vi "AddUser.vi"() -> ()   [LabVIEW 2020]
uses:
  <vilib>/Utility/error.llb/DialogType.ctl
  Global1.vi
  <vilib>/addons/database/Connection.llb/DB Tools Open Connec (String).vi
  <vilib>/addons/database/Connection.llb/Conn Execute.vi
  <vilib>/addons/database/Recordset.llb/Rec Destroy - Connection.vi
  <vilib>/addons/database/NI_Database_API.lvlib
panel:
  in  "员工编号":string
  in  "显示密码":bool
  in  "重复密码":string
  in  "权      限":enum16{"操作员", "管理员"}(ring)
  in  "取消":bool
  in  "确定":bool
  in  "密      码":string
  in  "用 户 名":string
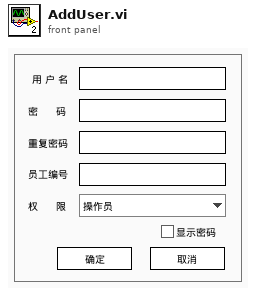
[diagram p1: front panel]
types:
  T1 = typedef "DialogType.ctl" = u16
  T2 = typedef "NI_Database_API.lvlib/Conn ObjectReference.ctl" = refnum<k1>
  T3 = typedef "NI_Database_API.lvlib/Rec ObjectReference.ctl" = refnum<k1>
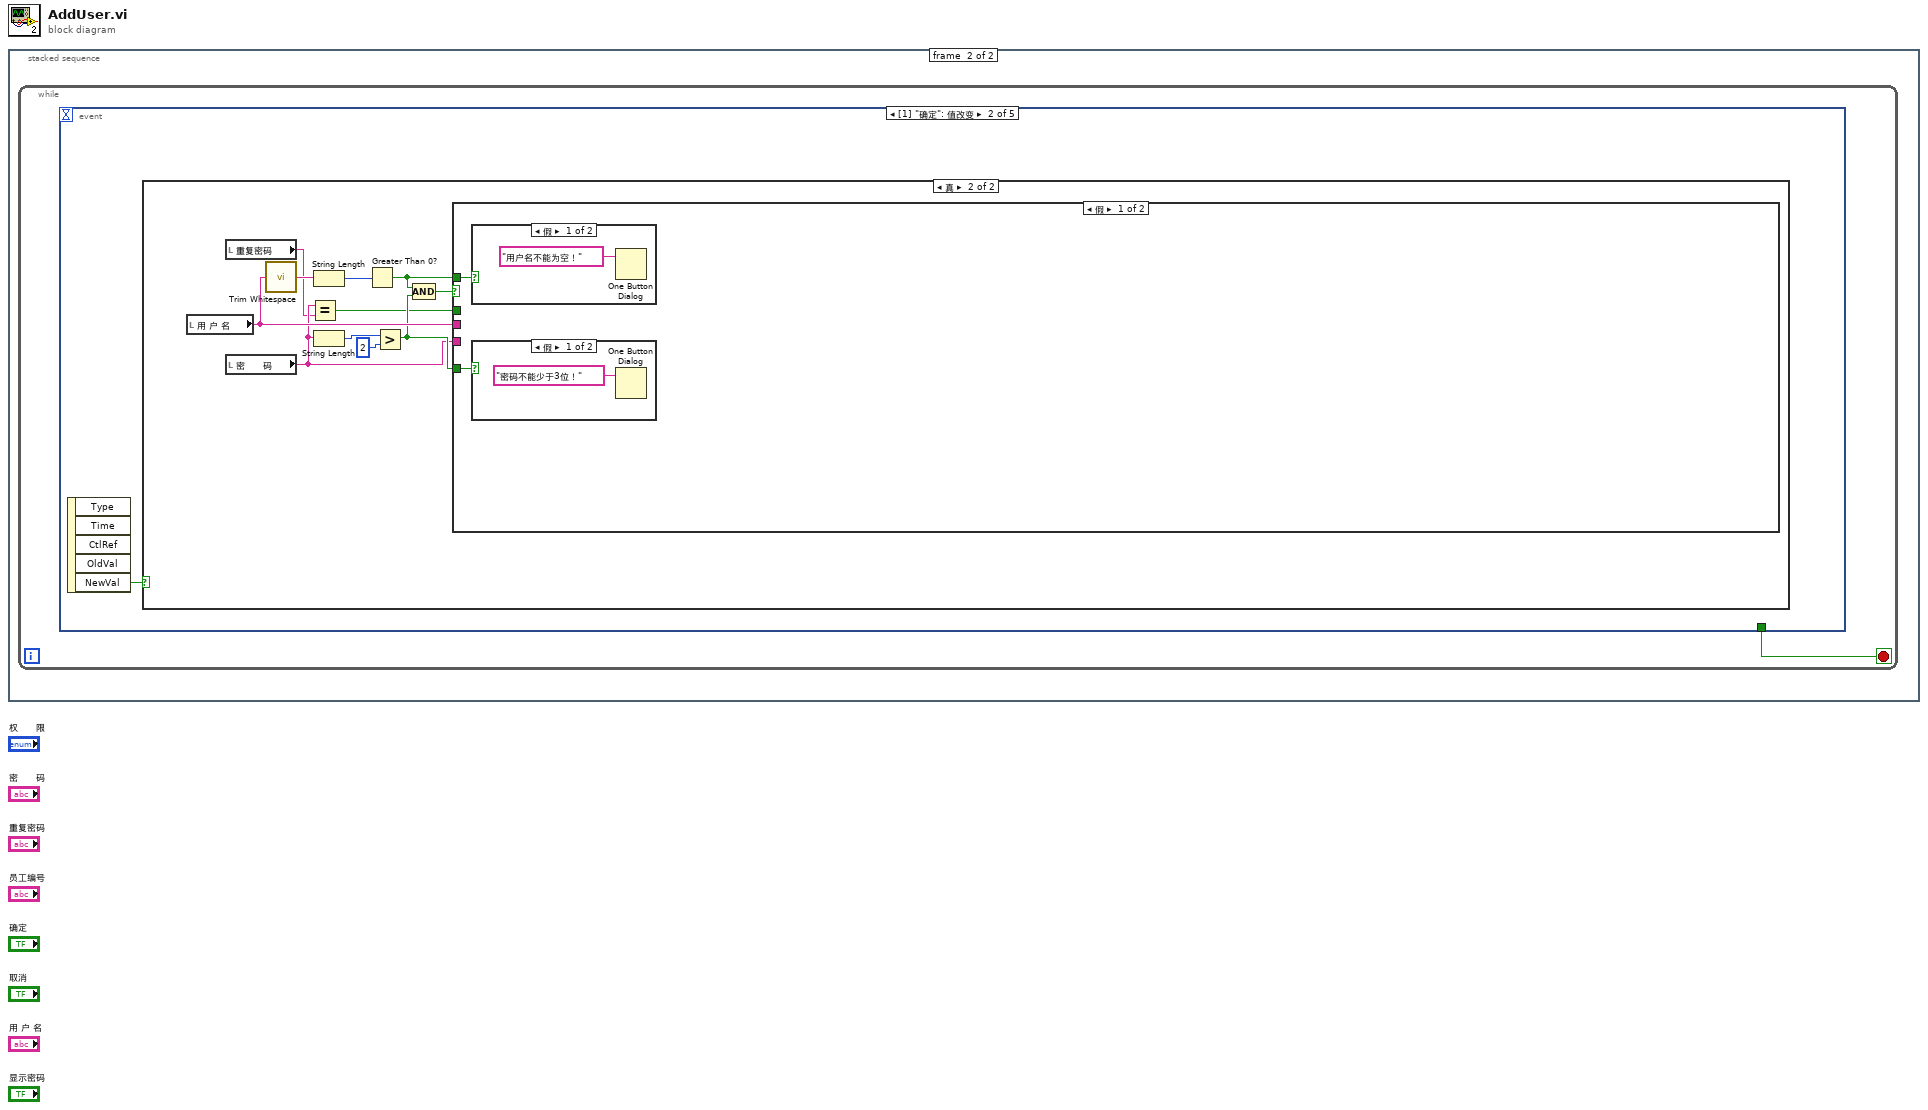
[diagram p0: block diagram]
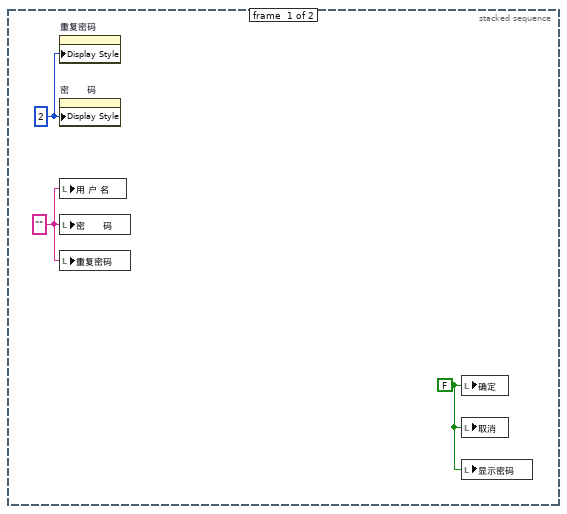
[diagram p2: hidden frame]
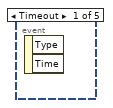
[diagram p3: hidden frame]
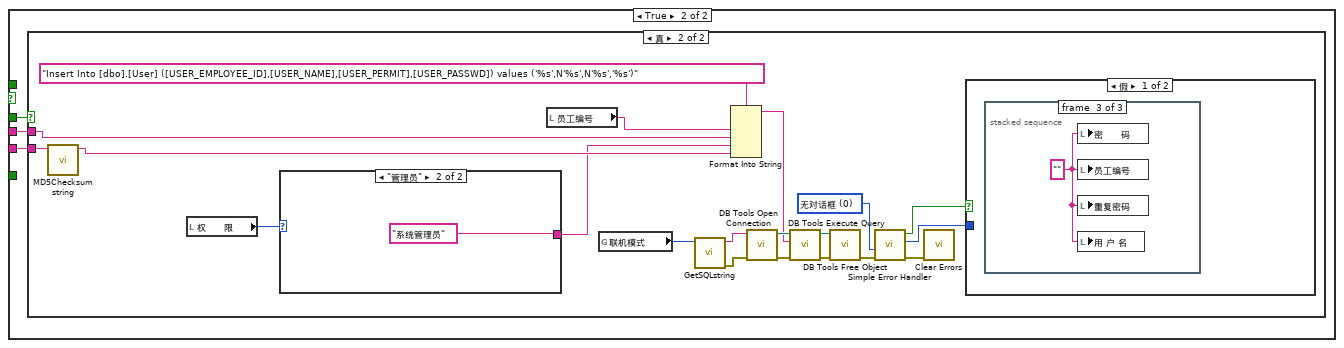
[diagram p7: hidden frame]
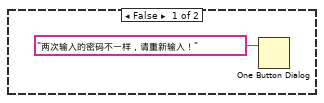
[diagram p8: hidden frame]
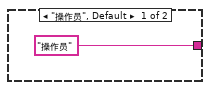
[diagram p9: hidden frame]
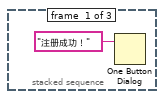
[diagram p10: hidden frame]
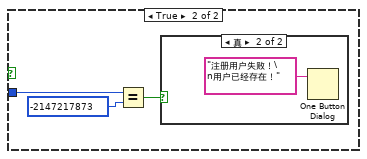
[diagram p12: hidden frame]
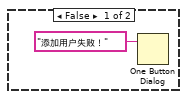
[diagram p13: hidden frame]
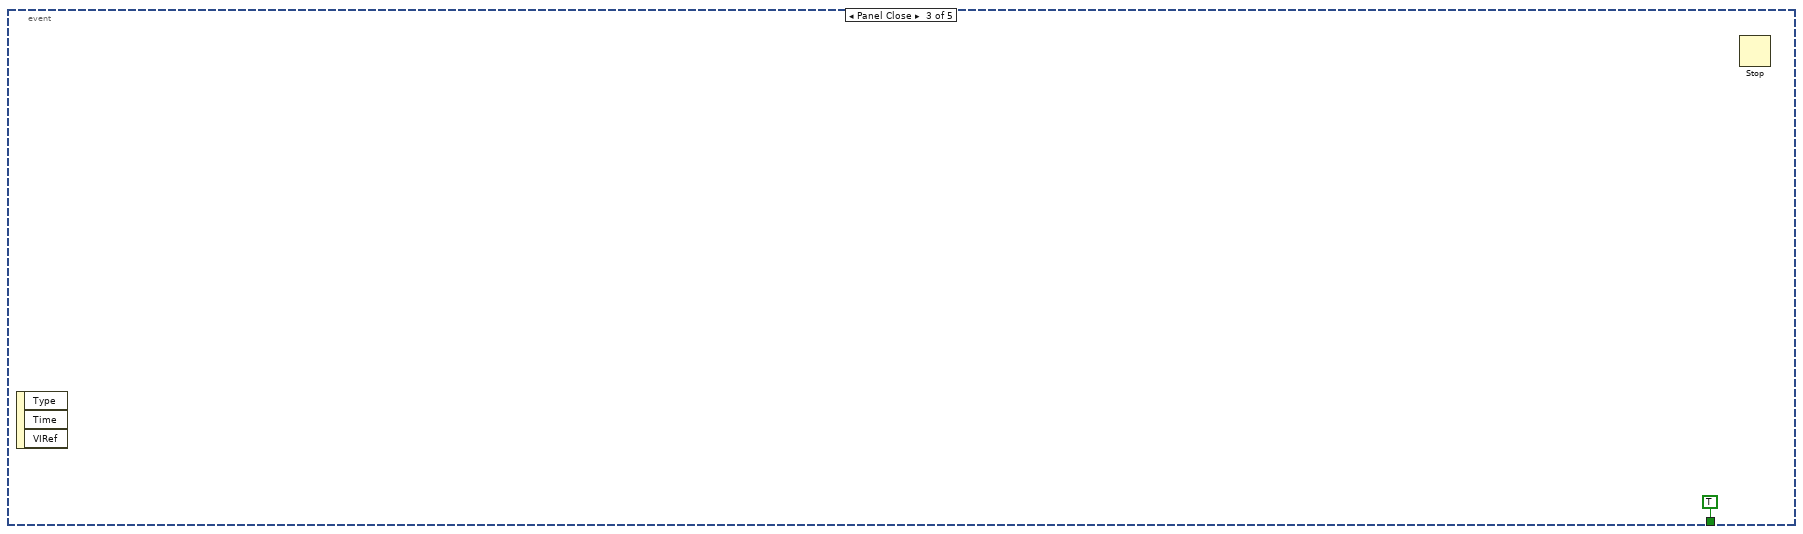
[diagram p14: hidden frame]
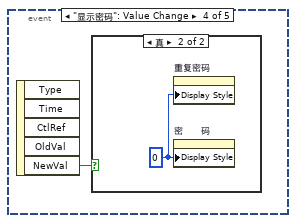
[diagram p15: hidden frame]
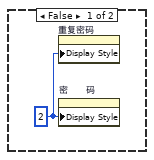
[diagram p16: hidden frame]
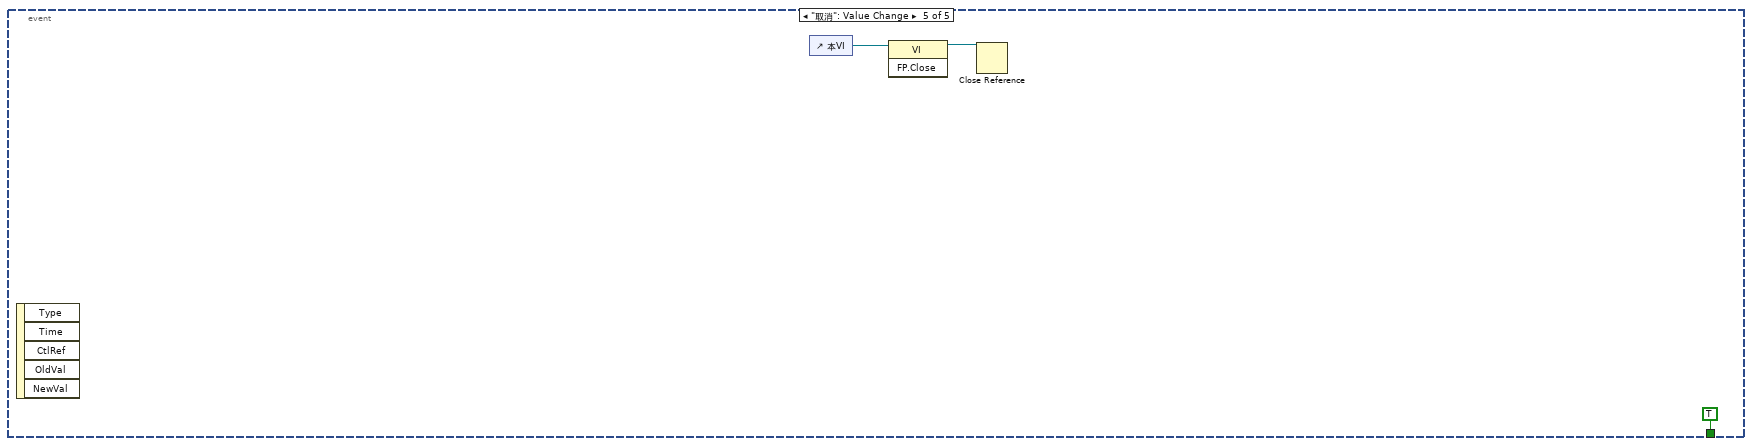
[diagram p17: hidden frame]
diagram:
  n1 = stacked-sequence {
    frame #0 {
      w1 = FALSE ("确定")
      w2 = u32 2 ("显示样式")
      w3 = ""
      n2 = property on="重复密码" class="Str"("Display Style"=w2) -> ()  [unwired: 2 in, 2 out]
      n3 = property on="密      码" class="Str"("Display Style"=w2) -> ()  [unwired: 2 in, 2 out]
      n4 = local write "用 户 名"(w3) -> ()
      n5 = local write "密      码"(w3) -> ()
      n6 = local write "重复密码"(w3) -> ()
      n7 = local write "确定"(w1) -> ()
      n8 = local write "取消"(w1) -> ()
      n9 = local write "显示密码"(w1) -> ()
    }
    frame #1 {
      n10 = while {
        stop <- w4 stop-if-true
        n11 = event shown="[1] \"确定\": 值改变" {
          selector: _ -> [_ _ _ _ _]
          dyn-events: _ -> [_ _ _ _ _]
          timeout: _ -> [_ _ _ _ _]
          tunnel: [_ _ TRUE _ TRUE] -> w4
          event Timeout {
            n12 = event-data() -> ()  [unwired: 1 in, 2 out]
          }
          event "确定": Value Change {
            n13 = event-data() -> ("NewVal"=w5:bool)  [unwired: 1 in, 4 out]
            n14 = case shown="真" w5 {
              frame False {
              }
              frame True {
                n15 = local read "用 户 名"() -> (w16:string)
                n16 = local read "重复密码"() -> (w7:string)
                n17 = local read "密      码"() -> (w8:string)
                n18 = call <vilib>:"Trim Whitespace.vi"("string"=w16) -> ("trimmed string"=w15:string)  [unwired: 1 in]
                n19 = Equal?(x=w8, y=w7) -> (x = y?=w6:bool)
                n20 = String Length(string=w15) -> (length=w14:i32)
                n21 = String Length(string=w8) -> (length=w13:i32)
                n22 = Greater Than 0?(x=w14) -> (x > 0?=w10:bool)
                n23 = Greater?(x=w13, y=2) -> (0:w9:bool)
                n24 = Compound Arithmetic op=AND(w10, w9) -> (w11:bool)
                n25 = case shown="假" w11 {
                  tunnel: w16 -> [_ w23]
                  tunnel: w8 -> [_ w22]
                  tunnel: w10 -> [w18 _]
                  tunnel: w9 -> [w17 _]
                  tunnel: w6 -> [_ w21]
                  frame False {
                    n26 = case shown="假" w18 {
                      frame False {
                        n27 = One Button Dialog(message="用户名不能为空！" ("消息")) -> ()  [unwired: 1 in, 1 out]
                      }
                      frame True {
                      }
                    }
                    n28 = case shown="假" w17 {
                      frame False {
                        n29 = One Button Dialog(message="密码不能少于3位！" ("消息")) -> ()  [unwired: 1 in, 1 out]
                      }
                      frame True {
                      }
                    }
                  }
                  frame True {
                    n30 = case shown="真" w21 {
                      tunnel: w23 -> [_ w35]
                      tunnel: w22 -> [_ w42]
                      frame False {
                        n31 = One Button Dialog(message="两次输入的密码不一样，请重新输入！" ("消息")) -> ()  [unwired: 1 in, 1 out]
                      }
                      frame True {
                        w41 = T1 0 items=["无对话框", "确定信息", "继续或停止信息", "确定信息＋警告", "继续/停止+警告"] ("type of dialog (OK msg:1)")
                        n32 = call <vilib>:"MD5Checksum string.vi"("Message String"=w42) -> ("MD5 message-digest"=w33:string)  [unwired: 10 in]
                        n33 = local read "权      限"() -> (w32:enum16{"操作员", "管理员"})
                        n34 = case shown="\"管理员\"" w32 {
                          tunnel: ["操作员" "系统管理员"] -> w31
                          frame "操作员", Default {
                          }
                          frame "管理员" {
                          }
                        }
                        n35 = local read "员工编号"() -> (w34:string)
                        n36 = global read "Global1.vi" "联机模式"() -> (w25:enum16{"单机", "追溯"})
                        n37 = call "GetSQLstring.vi"("联机模式"=w25) -> ("错误输出"=w27:errorcluster, "连接字符串"=w26:string)  [unwired: 9 in]
                        n38 = Format Into String(format string="Insert Into [dbo].[User] ([USER_EMPLOYEE_ID],[USER_NAME],[USER_PERMIT],[USER_PASSWD]) values ('%s',N'%s',N'%s','%s')", w34, w35, w31, w33) -> (resulting string=w36:string)  [unwired: 2 in, 1 out]
                        n39 = call-poly <vilib>:"DB Tools Open Connection.vi"("error in (no error)"=w27, "connection information"=w26) -> ("error out"=w44:errorcluster, "connection reference"=w43:T2)  [unwired: 6 in]
                        n40 = call-poly <vilib>:"DB Tools Execute Query.vi"("error in (no error)"=w44, "SQL query"=w36, "connection reference"=w43) -> ("error out"=w30:errorcluster, "recordset reference"=w28:T3)  [unwired: 5 in]
                        n41 = call-poly <vilib>:"DB Tools Free Object.vi"("error in (no error)"=w30, "recordset reference"=w28) -> ("error out"=w29:errorcluster)  [unwired: 8 in, 1 out]
                        n42 = call <vilib>:"Simple Error Handler.vi"("type of dialog (OK msg:1)"=w41, "error in (no error)"=w29) -> ("error?"=w40:bool, "code out"=w38:i32, "error out"=w39:errorcluster)  [unwired: 3 in, 2 out]
                        n43 = call <vilib>:"Clear Errors.vi"("error in (no error)"=w39) -> ()  [unwired: 5 in, 2 out]
                        n44 = case shown="假" w40 {
                          tunnel: w38 -> [_ w50]
                          frame False {
                            n45 = stacked-sequence {
                              frame #0 {
                                n46 = One Button Dialog(message="注册成功！" ("消息")) -> ()  [unwired: 1 in, 1 out]
                              }
                              frame #1 {
                              }
                              frame #2 {
                                w48 = ""
                                n47 = local write "密      码"(w48) -> ()
                                n48 = local write "员工编号"(w48) -> ()
                                n49 = local write "重复密码"(w48) -> ()
                                n50 = local write "用 户 名"(w48) -> ()
                              }
                            }
                          }
                          frame True {
                            n51 = Equal?(x=w50, y=-2147217873) -> (x = y?=w51:bool)
                            n52 = case shown="真" w51 {
                              frame False {
                                n53 = One Button Dialog(message="添加用户失败！" ("消息")) -> ()  [unwired: 1 in, 1 out]
                              }
                              frame True {
                                n54 = One Button Dialog(message="注册用户失败！\n用户已经存在！" ("消息")) -> ()  [unwired: 1 in, 1 out]
                              }
                            }
                          }
                        }
                      }
                    }
                  }
                }
              }
            }
          }
          event Panel Close {
            n55 = event-data() -> ()  [unwired: 1 in, 3 out]
            n56 = Stop() -> ()  [unwired: 1 in]
          }
          event "显示密码": Value Change {
            n57 = event-data() -> ("NewVal"=w55:bool)  [unwired: 1 in, 4 out]
            n58 = case shown="真" w55 {
              frame False {
                w56 = u32 2 ("显示样式")
                n59 = property on="重复密码" class="Str"("Display Style"=w56) -> ()  [unwired: 2 in, 2 out]
                n60 = property on="密      码" class="Str"("Display Style"=w56) -> ()  [unwired: 2 in, 2 out]
              }
              frame True {
                w57 = u32 0 ("显示样式")
                n61 = property on="重复密码" class="Str"("Display Style"=w57) -> ()  [unwired: 2 in, 2 out]
                n62 = property on="密      码" class="Str"("Display Style"=w57) -> ()  [unwired: 2 in, 2 out]
              }
            }
          }
          event "取消": Value Change {
            n63 = event-data() -> ()  [unwired: 1 in, 5 out]
            n64 = control-ref of="本VI"() -> (w59:refnum<vi>)
            n65 = invoke class="VI" method="FP.Close"(reference=w59) -> (reference out=w58:refnum<vi>)  [unwired: 2 in, 2 out]
            n66 = Close Reference(reference=w58) -> ()  [unwired: 1 in, 1 out]
          }
        }
      }
    }
  }
